vi "Receive - UDP (CommPort).vi"() -> ()   [LabVIEW 2020]
uses:
  src/_controls/comm_verification_rx.ctl
  src/_controls/comm_udp_rx.ctl
  src/_polimorphicInstances/session/Fdx Create Session (Rx-VL-Oriented).vi
  src/bsp/AFDX_Receive/Fdx Create Rx VL.vi
  src/_polimorphicInstances/udpPort/Fdx Create UDP Port (RX-CommPort).vi
  src/_polimorphicInstances/control/Fdx Start (Rx).vi
  src/_polimorphicInstances/control/Fdx Stop (Rx).vi
  src/_polimorphicInstances/session/Fdx Close Session (Port).vi
  src/AIM664LV.lvlib
panel:
  out "current irig time":T1={"SignOut"=40, "DayOut"=1, "HourOut"=1, "MinOut"=28, "SecondOut"=39, "MilliSecOut"=539, "MicroSecOut"=300, "NanoSecOut"=0, "InfoOut"=0, "Mode"=3}
  in  "CommPort Config":T2={"PortType"=enum."FDX_UDP_SAMPLING", "SubVIId"=1, "domainID"=1, "sideID"=1, "locationID"=1, "partitionID"=1, "UdpSrcPort"=12345, "UdpDstPort"=12346, "UdpNumBufMessages"=0, "UdpMaxMessageSize"=1000, "UdpSamplingRate"=0} {"partitionID" format="%.0b"}
  out "BytesRead":u32
  out "Data":u8[](array[numeric])=[1, 2, 3, 4, 0, 0, 0, 0, 0, 0, 0, 0, 0, 0, 0, 0, 0, 0, 0, 0, 0, 0, 0, 0, 0, 0, 0, 0, 0, 0, 0, 0, 0, 0, 0, 0, 0, 0, 0, 0, 0, 0, 0, 0, 0, 0, 0, 0, 0, 0, 0, 0, 0, 0, 0, 0, 0, 0, 0, 0, 0, 0, 0, 0, 0, 0, 0, 0, 0, 0, 0, 0, 0, 0, 0, 0, 0, 0, 0, 0, 0, 0, 0, 0, 0, 0, 0, 0, 0, 0, 0, 0, 0, 0, 0, 0, 0, 0, 0, 0] format="%.0x"
  in  "Messages to Read (1)":u32=1
  in  "VL Config":T3={"VlId"=60, "VLRange"=2, "VerificationMode"=0, "Bag"=0, "Jitter"=0, "MaxFrameLength"=0, "MaxSkew"=0, "VLBufSize"=32768, "FilterMode"=0, "FilterPosition"=0, "Padding"=0, "FilterMask"=0, "FilterData"=0, "MinFrameLength"=0} {"FilterMode" items=["FDX_RX_VL_FLT_DIS", "FDX_RX_VL_FLT_ENA ", "FDX_RX_VL_FLT_ENA_INV"]; "MaxFrameLength" format="%.0x"; "VerificationMode" items=["FDX_RX_VL_CHECK_ENA_DEFAULT"=65535, "FDX_RX_VL_CHECK_REDMAM"=16, "DX_RX_VL_CHECK_TRAFIC"=8, "FDX_RX_VL_CHECK_FRAMESIZE"=4, "FDX_RX_VL_CHECK_SNINTEG"=2, "FDX_RX_VL_CHECK_INVPAC"=1, "FDX_RX_VL_CHECK_DISA"=0]}
  out "PortInitOut":T4={"PortConfig"=0, "PortUsed"=1, "GlobalMemFree"=0, "SharedMemFree"=0} {"PortConfig" items=["FDX_SINGLE", "FDX_REDUNDANT"]}
  in  "Port":u32=1
  in  "Board":u32
  in  "Period mS":u32=200
  out "error out":errorcluster
  in  "stop":bool
  out "current time":timestamp
  # "ARINC 664 - Receiving through UDP with Communication Port"
  # "Overview: Setup the board to transmit package as raw frames.\nRequirement: One AIM ARINC-664 board with installed AIM ARINC 664 BSP.\nRestrictions: None.\nInstruction:\n1. Select the Board ID (0 if you have only one board in your system) and the port number. If you want to validate between two ports in one device, you can use tx board and Rx Board\n2. Run the VI.\n3. See the result in Current IRIG Time"
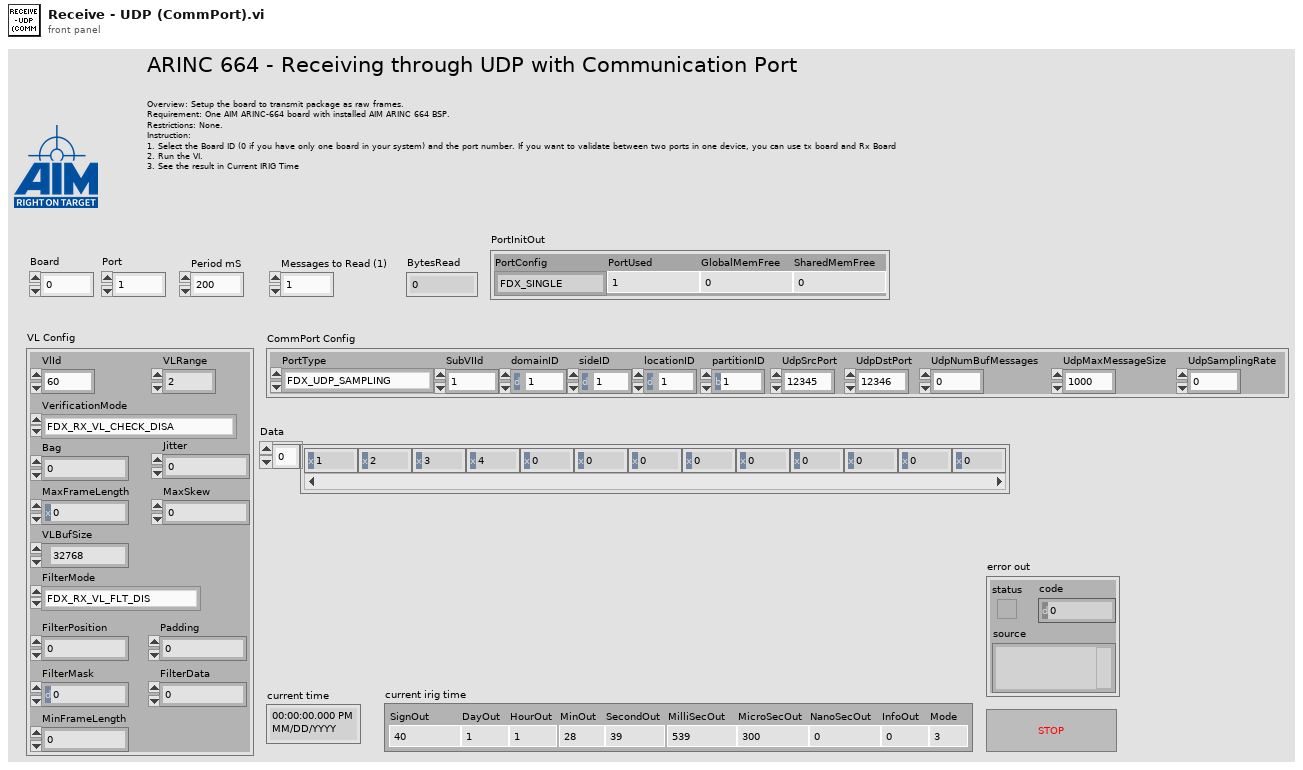
[diagram p1: front panel]
types:
  T1 = cluster{"SignOut":i32, "DayOut":u32, "HourOut":u32, "MinOut":u32, "SecondOut":u32, "MilliSecOut":u32, "MicroSecOut":u32, "NanoSecOut":u32, "InfoOut":u32, "Mode":u32}
  T2 = typedef "AIM664LV.lvlib/comm_udp_rx.ctl" = cluster{"PortType":enum16{"FDX_UDP_SAMPLING", "FDX_UDP_QUEUING"}, "SubVIId":u32, "domainID":u8, "sideID":u8, "locationID":u8, "partitionID":u8, "UdpSrcPort":u16, "UdpDstPort":u16, "UdpNumBufMessages":u32, "UdpMaxMessageSize":u32, "UdpSamplingRate":u32}
  T3 = typedef "AIM664LV.lvlib/comm_verification_rx.ctl" = cluster{"VlId":u16, "VLRange":u32, "VerificationMode":u32, "Bag":u32, "Jitter":u32, "MaxFrameLength":u32, "MaxSkew":u32, "VLBufSize":u32, "FilterMode":u32, "FilterPosition":u32, "Padding":u32, "FilterMask":u32, "FilterData":u32, "MinFrameLength":u32}
  T4 = cluster{"PortConfig":u32, "PortUsed":u32, "GlobalMemFree":u32, "SharedMemFree":u32}
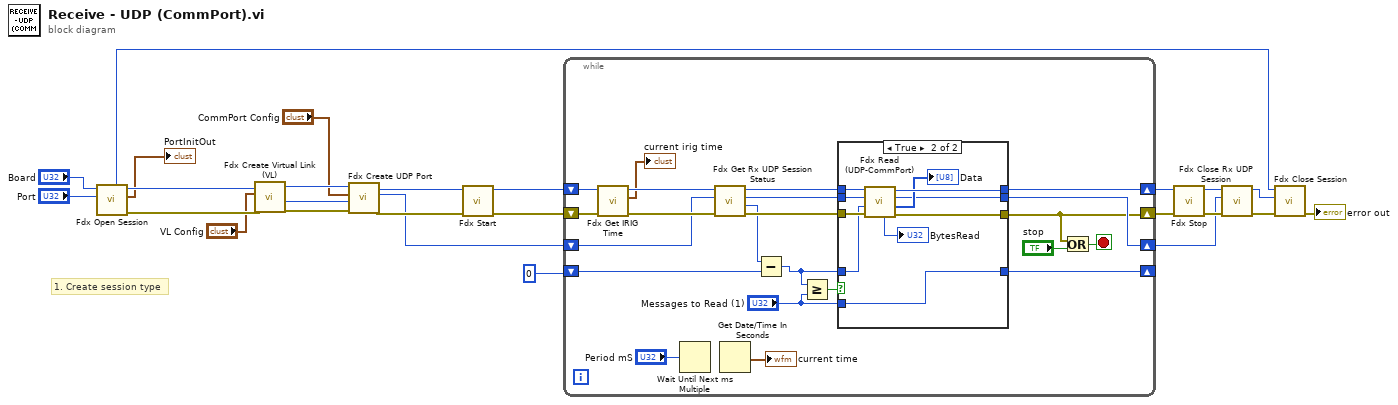
[diagram p0: block diagram]
diagram:
  # "1. Create session type"
  n1 = call-poly "Fdx Open Session.vi"("port"="Port", "board"="Board") -> ("error out"=w24:errorcluster, "PortInitOut"=→"PortInitOut":T4, "InstrumentHandle_port out"=w25:u32, "InstrumentHandle_board out"=w5:u32)  [unwired: 4 in, 2 out]
  n2 = call-poly "Fdx Create Virtual Link (VL).vi"("error in (no error)"=w24, "VL Config"="VL Config", "InstrumentHandle_port in"=w25) -> ("error out"=w22:errorcluster, "VlId"=w8:u16, "InstrumentHandle_port out"=w23:u32)  [unwired: 6 in]
  n3 = call-poly "Fdx Create UDP Port.vi"("error in (no error)"=w22, "VlId"=w8, "CommPort Config"="CommPort Config", "port handle in"=w23) -> ("error out"=w20:errorcluster, "commPort handle out"=w17:u32, "port handle out"=w21:u32)  [unwired: 4 in, 1 out]
  n4 = call-poly "Fdx Start.vi"("error in (no error)"=w20, "InstrumentHandle_port in"=w21) -> ("error out"=w2:errorcluster, "InstrumentHandle_port out"=w19:u32)  [unwired: 8 in]
  n5 = while {
    shift-right: [w40] -> w18
    shift-left: w19 -> [w36]
    shift-right: [w37] -> w3
    shift-left: w17 -> [w27]
    shift-right: [w41] -> _
    shift-left: u32 0 ("MsgCount") -> [w46]
    shift-right: [w28] -> w1
    shift-left: w2 -> [w31]
    stop <- w30 stop-if-true
    n6 = call "Fdx Get IRIG Time.vi"("error in (no error)"=w31, "InstrumentHandle_board in"=w36) -> ("error out"=w35:errorcluster, "Curent Irig Time"=→"current irig time":T1, "InstrumentHandle_board out"=w34:u32)  [unwired: 7 in]
    n7 = Wait Until Next ms Multiple(millisecond multiple="Period mS") -> ()  [unwired: 1 out]
    n8 = call "Fdx Get Rx UDP Session Status.vi"("error in (no error)"=w35, "UdpHandle in"=w27, "InstrumentHandle_port in"=w34) -> ("error out"=w45:errorcluster, "MsgCount"=w38:u32, "UdpHandle out"=w39:u32, "InstrumentHandle_port out"=w44:u32)  [unwired: 4 in, 1 out]
    n9 = Get Date/Time In Seconds() -> (seconds since 1Jan1904=→"current time":timestamp)
    n10 = Subtract(x=w38, y=w46) -> (x-y=w26:u32)
    n11 = Greater Or Equal?(x=w26, y="Messages to Read (1)") -> (x >= y?=w43:bool)
    n12 = case shown="True" w43 {
      tunnel: w45 -> [w49 w59]
      tunnel: w44 -> [w51 w60]
      tunnel: "Messages to Read (1)" -> [_ w61]
      tunnel: [w51 w58] -> w40
      tunnel: w26 -> [w50 w54]
      tunnel: [w50 w61] -> w41
      tunnel: [w49 w57] -> w28
      tunnel: w39 -> [w48 w55]
      tunnel: [w48 w52] -> w37
      frame False {
      }
      frame True {
        n13 = call "Fdx Read (UDP-CommPort).vi"("error in (no error)"=w59, "MsgCount(1)"=w54, "UdpHandle in"=w55, "InstrumentHandle_port in"=w60) -> ("error out"=w57:errorcluster, "Data"=→"Data":u8[], "UdpHandle out"=w52:u32, "InstrumentHandle_port out"=w58:u32, "MsgRead"=→"BytesRead":u32)  [unwired: 3 in]
      }
    }
    n14 = Or(x=w28, y="stop") -> (x .or. y?=w30:bool)
  }
  n15 = call-poly "Fdx Stop.vi"("error in (no error)"=w1, "InstrumentHandle_port in"=w18) -> ("error out"=w16:errorcluster, "InstrumentHandle_port out"=w4:u32)  [unwired: 8 in]
  n16 = call "Fdx Close Rx UDP Session.vi"("error in (no error)"=w16, "UdpHandle in"=w3, "InstrumentHandle_port in"=w4) -> ("error out"=w15:errorcluster, "InstrumentHandle_port out"=w6:u32)  [unwired: 7 in]
  n17 = call-poly "Fdx Close Session.vi"("error in (no error)"=w15, "InstrumentHandle_port in"=w6, "InstrumentHandle_board in"=w5) -> ("error out"=→"error out":errorcluster)  [unwired: 8 in]
